vi "is abstract node.vi"(8 "error in":errorcluster, 11 "Asynchronous Module Editor Node in":refnum<class "Asynchronous Module Editor Node.lvclass">) -> (0 "error out":errorcluster, 2 "abstract":bool, 3 "Asynchronous Module Editor Node out":refnum<class "Asynchronous Module Editor Node.lvclass">)   [LabVIEW 2013, in "Asynchronous Module Editor Node.lvclass"]
uses:
  Asynchronous Module Editor Node.lvclass
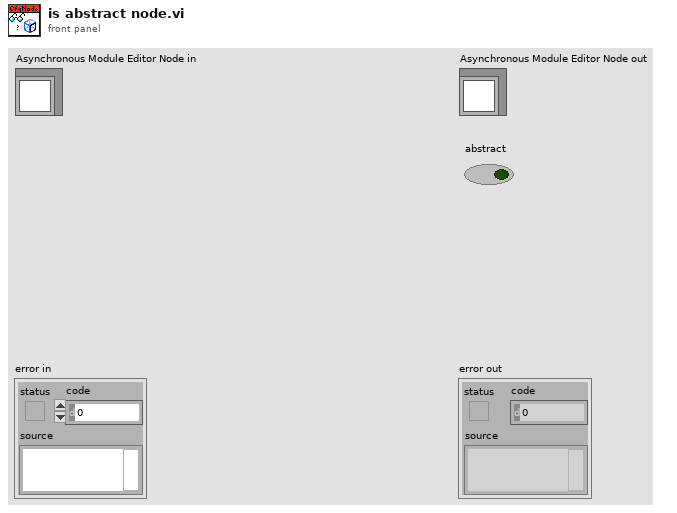
[diagram p1: front panel]
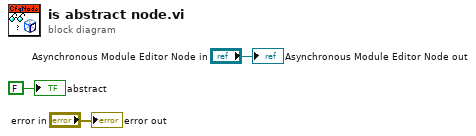
[diagram p0: block diagram]
diagram:
  "error out" <- "error in"
  "Asynchronous Module Editor Node out" <- "Asynchronous Module Editor Node in"
  "abstract" <- FALSE ("abstract")
